vi "Initialize Mover.vi"(7 "Mass (1)":dbl=1.0, 8 "error in":errorcluster, 9 "Location (0,0)":cluster{"X":dbl, "Y":dbl}, 10 "Velocity (0,0)":cluster{"X":dbl, "Y":dbl}, 11 "Acceleration (0,0)":cluster{"X":dbl, "Y":dbl}) -> (0 "error out":errorcluster, 3 "Mover out":refnum<class "Mover.lvclass">)   [LabVIEW 2016, in "Mover.lvclass"]
doc: "Initialized new Mover object with provided parameters"
uses:
  Mover.lvclass
  PVector/PVector.lvclass
  Mover.lvclass/Mover.ctl
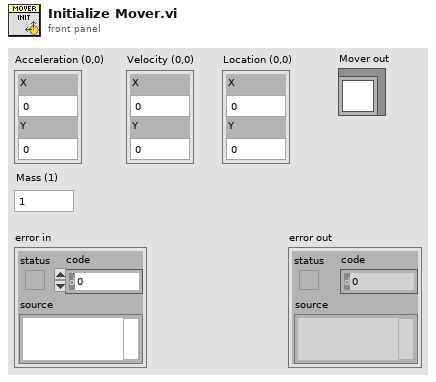
[diagram p1: front panel]
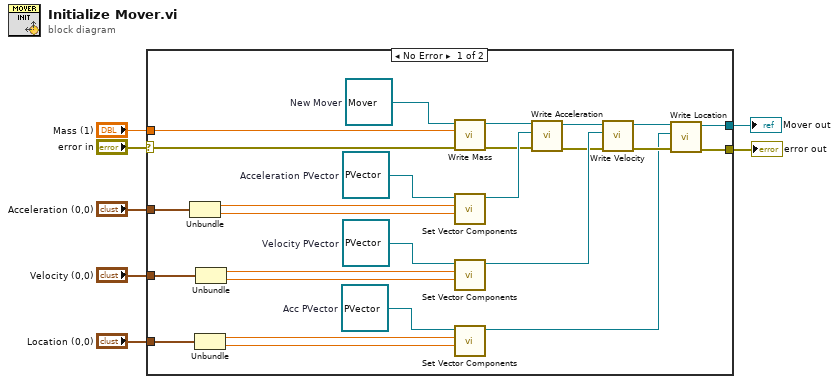
[diagram p0: block diagram]
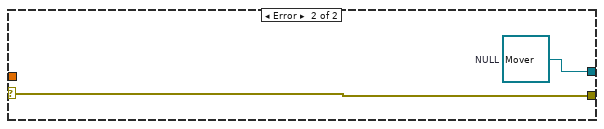
[diagram p2: hidden frame]
diagram:
  n1 = case shown="No Error" "error in" {
    selector: "error in" -> [w28 w35]
    tunnel: [w27 w35] -> w6
    tunnel: "Mass (1)" -> [w29 _]
    tunnel: [w26 w34] -> w4
    tunnel: "Acceleration (0,0)" -> [w16 _]
    tunnel: "Velocity (0,0)" -> [w13 _]
    tunnel: "Location (0,0)" -> [w10 _]
    frame No Error {
      w22 = refnum<class "PVector.lvclass"> refnum  # Acc PVector
      w23 = refnum<class "PVector.lvclass"> refnum  # Velocity PVector
      w25 = refnum<class "PVector.lvclass"> refnum  # Acceleration PVector
      w33 = refnum<class "Mover.lvclass"> refnum  # New Mover
      n2 = Unbundle(w16) -> ("X"=w15:dbl, "Y"=w14:dbl)
      n3 = Unbundle(w10) -> ("X"=w9:dbl, "Y"=w8:dbl)
      n4 = Unbundle(w13) -> ("X"=w12:dbl, "Y"=w11:dbl)
      n5 = call "Write Mass.vi"("error in"=w28, "Mass"=w29, "Mover in"=w33) -> ("error out"=w21:errorcluster, "Mover out"=w32:refnum<class "Mover.lvclass">)  [unwired: 7 in]
      n6 = call "Set Vector Components.vi"("Y"=w14, "X"=w15, "PVector in"=w25) -> ("PVector out"=w24:refnum<class "PVector.lvclass">)  [unwired: 7 in, 1 out]
      n7 = call "Set Vector Components.vi"("Y"=w11, "X"=w12, "PVector in"=w23) -> ("PVector out"=w20:refnum<class "PVector.lvclass">)  [unwired: 7 in, 1 out]
      n8 = call "Set Vector Components.vi"("Y"=w8, "X"=w9, "PVector in"=w22) -> ("PVector out"=w17:refnum<class "PVector.lvclass">)  [unwired: 7 in, 1 out]
      n9 = call "Write Acceleration.vi"("error in"=w21, "Acceleration PVector"=w24, "Mover in"=w32) -> ("error out"=w19:errorcluster, "Mover out"=w31:refnum<class "Mover.lvclass">)  [unwired: 7 in]
      n10 = call "Write Velocity.vi"("error in"=w19, "Velocity PVector"=w20, "Mover in"=w31) -> ("error out"=w18:errorcluster, "Mover out"=w30:refnum<class "Mover.lvclass">)  [unwired: 7 in]
      n11 = call "Write Location.vi"("error in"=w18, "Location PVector"=w17, "Mover in"=w30) -> ("error out"=w27:errorcluster, "Mover out"=w26:refnum<class "Mover.lvclass">)  [unwired: 7 in]
    }
    frame Error {
      w34 = refnum<class "Mover.lvclass"> refnum  # NULL
    }
  }
  "error out" <- w6
  "Mover out" <- w4
